vi "COMTRADE Write Data.vi"   [LabVIEW 2012, in "NI_EP_COMTRADE.lvlib"]
doc: "Writes configuration information and data to the specified .cfg and .dat files. You must set <B>open mode</B> to Create or Create or replace in the COMTRADE Open VI to open files. Otherwise this VI returns an error."
uses:
  <vilib>/addons/Electrical Power/File IO/NI_EP_COMTRADE.lvlib
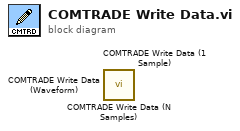
[diagram p0: block diagram]
diagram:
  n1 = call <vilib>:"COMTRADE Write Data (N Samples).vi"() -> ()  [unwired: 10 in, 2 out]
  n2 = call <vilib>:"COMTRADE Write Data (1 Sample).vi"() -> ()  [unwired: 10 in, 2 out]
  n3 = call <vilib>:"COMTRADE Write Data (Waveform).vi"() -> ()  [unwired: 10 in, 2 out]
